vi "ManageQ.vi"(7 "QStateIn":T1(ring), 8 "Error In":errorcluster, 9 "State In":string="Message In", 11 "QueueRefIn":refnum<queue>) -> (0 "Error Out":errorcluster, 2 "State Out":string, 3 "QueueRefOut":refnum<queue>)   [LabVIEW 2024]
doc: "<b>Functionality of the VI</b>\n\nThis VI manage the queue operation to execute the application"
panel:
  # "Outputs to the VI"
  # "Inputs to the VI"
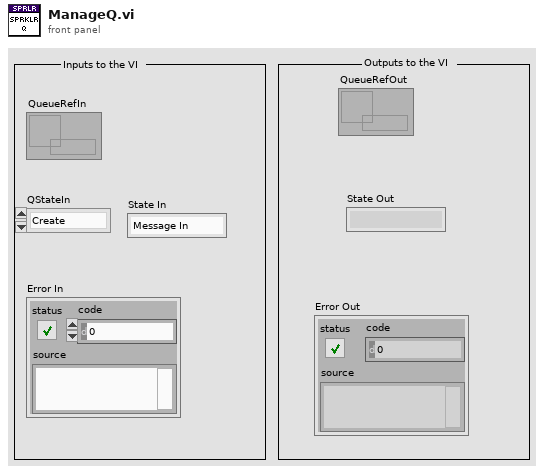
[diagram p1: front panel]
types:
  T1 = enum16{"Create", "Enqueue", "Dequeue", "Enstack", "Flush", "Release"}
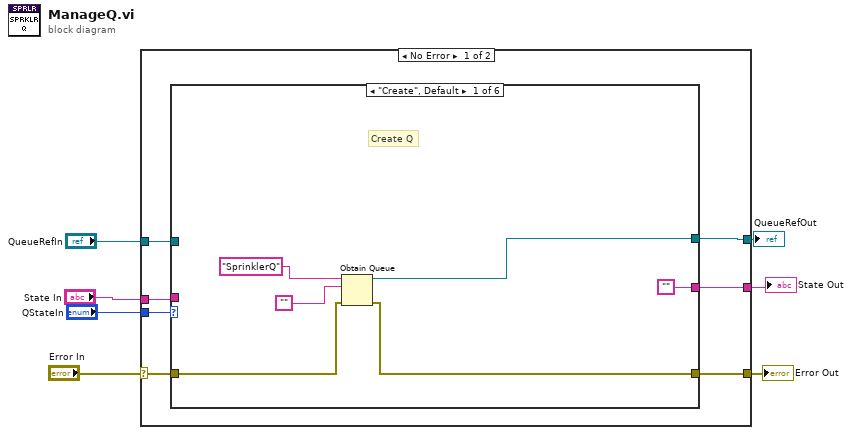
[diagram p0: block diagram]
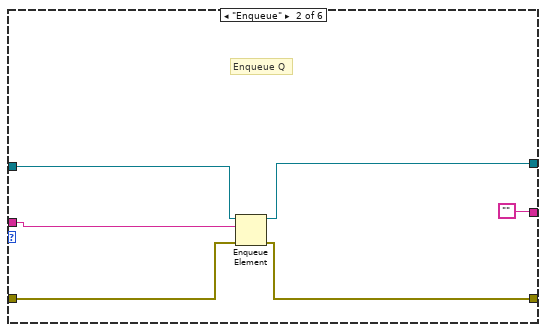
[diagram p2: hidden frame]
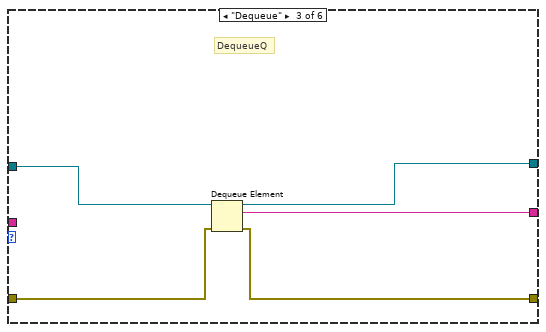
[diagram p3: hidden frame]
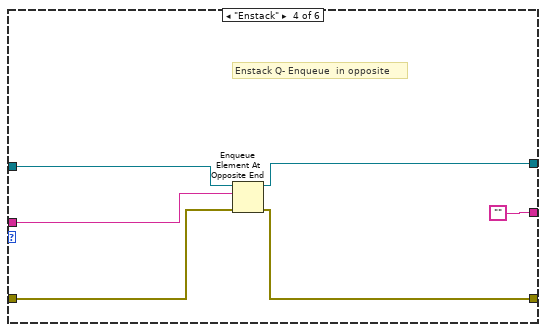
[diagram p4: hidden frame]
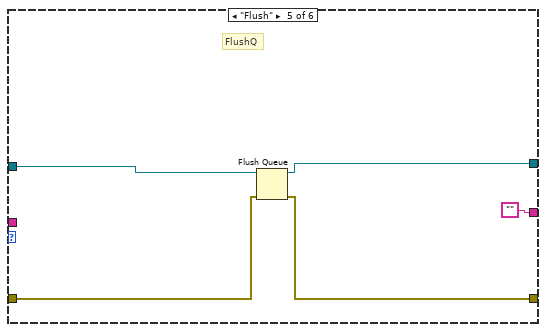
[diagram p5: hidden frame]
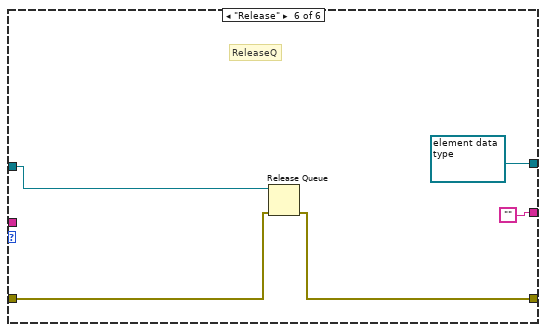
[diagram p6: hidden frame]
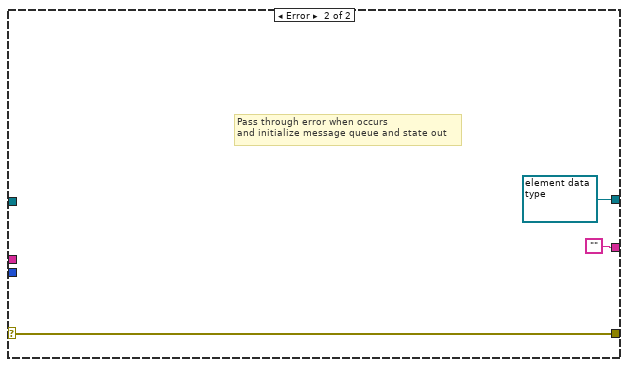
[diagram p7: hidden frame]
diagram:
  n1 = case shown="No Error" "Error In" {
    selector: "Error In" -> [w13 w48]
    tunnel: "QStateIn" -> [w14 _]
    tunnel: [w12 w48] -> w5
    tunnel: "State In" -> [w11 _]
    tunnel: [w10 ""] -> w3
    tunnel: [w9 refnum<queue> refnum ("queue out 2")] -> w2
    tunnel: "QueueRefIn" -> [w8 _]
    frame No Error {
      n2 = case shown="\"Create\", Default" w14 {
        tunnel: w13 -> [w20 w26 w31 w37 w41 w47]
        tunnel: [w19 w25 w30 w34 w40 w46] -> w12
        tunnel: [w18 w23 w28 w36 w42 refnum<queue> refnum ("queue out")] -> w9
        tunnel: w11 -> [_ w24 _ w35 _ _]
        tunnel: ["" ("element data type") "" ("element data type") w29 "" ("element data type") "" ("element data type") "" ("element data type")] -> w10
        tunnel: w8 -> [_ w21 w27 w32 w38 w43]
        frame "Create", Default {
          # "Create Q"
          n3 = Obtain Queue(name (unnamed)="SprinklerQ" ("QName"), element data type="", error in (no error)=w20) -> (queue out=w18:refnum<queue>, error out=w19:errorcluster)  [unwired: 2 in, 1 out]
        }
        frame "Enqueue" {
          # "Enqueue Q"
          n4 = Enqueue Element(queue=w21, element=w24, error in (no error)=w26) -> (queue out=w23:refnum<queue>, error out=w25:errorcluster)  [unwired: 1 in, 1 out]
        }
        frame "Dequeue" {
          # "DequeueQ"
          n5 = Dequeue Element(queue=w27, error in (no error)=w31) -> (queue out=w28:refnum<queue>, element=w29:string, error out=w30:errorcluster)  [unwired: 1 in, 1 out]
        }
        frame "Enstack" {
          # "Enstack Q- Enqueue  in opposite"
          n6 = Enqueue Element At Opposite End(queue=w32, element=w35, error in (no error)=w37) -> (queue out=w36:refnum<queue>, error out=w34:errorcluster)  [unwired: 1 in, 1 out]
        }
        frame "Flush" {
          # "FlushQ"
          n7 = Flush Queue(queue=w38, error in (no error)=w41) -> (queue out=w42:refnum<queue>, error out=w40:errorcluster)  [unwired: 1 out]
        }
        frame "Release" {
          # "ReleaseQ"
          n8 = Release Queue(queue=w43, error in (no error)=w47) -> (error out=w46:errorcluster)  [unwired: 1 in, 2 out]
        }
      }
    }
    frame Error {
      # "Pass through error when occurs\nand initialize message queue and state out"
    }
  }
  "Error Out" <- w5
  "State Out" <- w3
  "QueueRefOut" <- w2
